vi "get request timeout.vi"(8 "error in (no error)":errorcluster, 11 "Nominal Client in":refnum<class "Nominal Client.lvclass">) -> (0 "error out":errorcluster, 2 "request timeout (ms)":i32, 3 "Nominal Client out":refnum<class "Nominal Client.lvclass">)   [LabVIEW 2020, in "Nominal Client.lvclass"]
uses:
  Nominal Client.lvclass
  Nominal Client.lvclass/Nominal Client.ctl
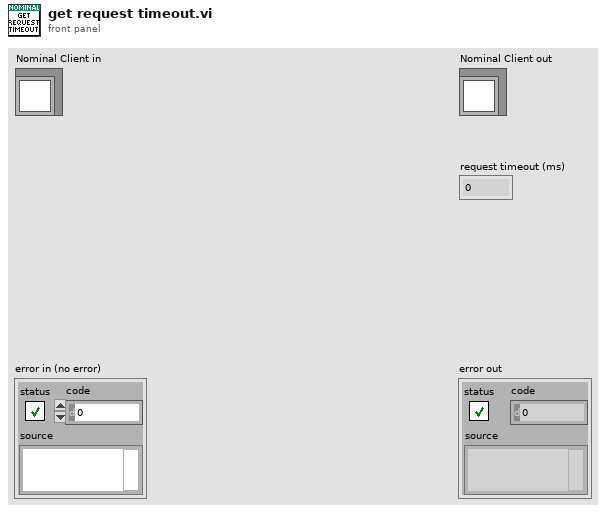
[diagram p1: front panel]
types:
  T1 = typedef "Nominal Client.lvclass/private_data.ctl" = cluster{"API Token":string, "workspace":refnum<class "workspace.lvclass">, "Available Workspaces":refnum<class "workspace.lvclass">[], "reqwest":refnum<class "reqwest.lvclass">, "timeout ms":i32}
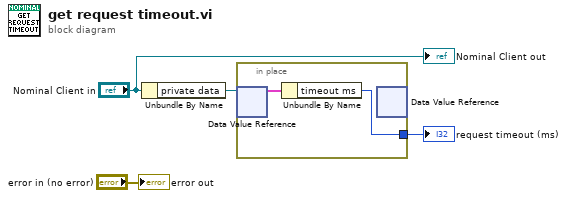
[diagram p0: block diagram]
diagram:
  n1 = Unbundle By Name("Nominal Client in") -> ("private data"=w1:refnum<data-value>)
  n2 = in-place {
    in-place-border: [w5] -> w2
    n3 = in-place-dvr #1(w1) -> (w6:T1)  [unwired: 1 out]
    n4 = Unbundle By Name(w6) -> ("timeout ms"=w5:i32)
    n5 = in-place-dvr #1() -> ()  [unwired: 1 in, 2 out]
  }
  "request timeout (ms)" <- w2
  "error out" <- "error in (no error)"
  "Nominal Client out" <- "Nominal Client in"
